vi "Evaluate Part 1.vi"() -> ()   [LabVIEW 2020]
uses:
  Descrambler/Descrambler.lvclass
panel:
  out "sum":i32=142
  in  "Input":string="1abc2\npqr3stu8vwx\na1b2c3d4e5f\ntreb7uchet"
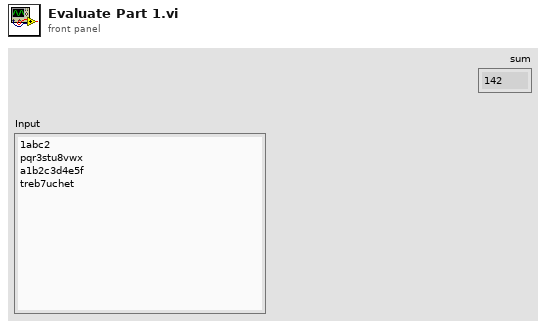
[diagram p1: front panel]
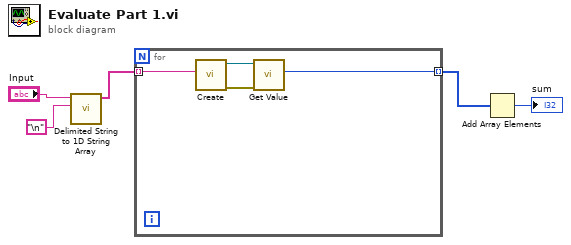
[diagram p0: block diagram]
diagram:
  n1 = call <vilib>:"Delimited String to 1D String Array.vi"("delimiter"="\n", "delimited string"="Input") -> ("string array"=w3:string[])  [unwired: 9 in]
  n2 = for {
    tunnel: w3 -> [w7] mode=indexing
    tunnel: [w6] -> w2 mode=indexing
    n3 = call "Create.vi"("String"=w7) -> ("error out"=w8:errorcluster, "Descrambler"=w9:refnum<class "Descrambler.lvclass">)  [unwired: 9 in]
    n4 = call "Get Value.vi"("error in (no error)"=w8, "Descrambler in"=w9) -> ("Value"=w6:i32)  [unwired: 7 in, 2 out]
  }
  n5 = Add Array Elements(numeric array=w2) -> (sum=→"sum":i32)
